vi "Determine Warnings.vi"() -> ()   [LabVIEW 2014]
panel:
  out "Warning Text":string
  out "Warning?":bool
  in  "Mininum Min Temp":dbl
  in  "Max Temp":dbl
  in  "Current Temp":dbl
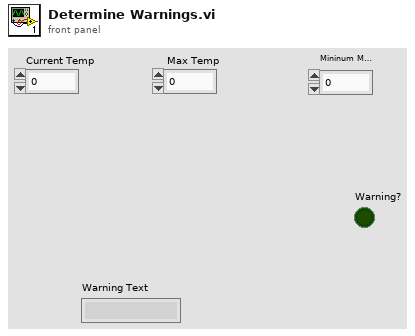
[diagram p1: front panel]
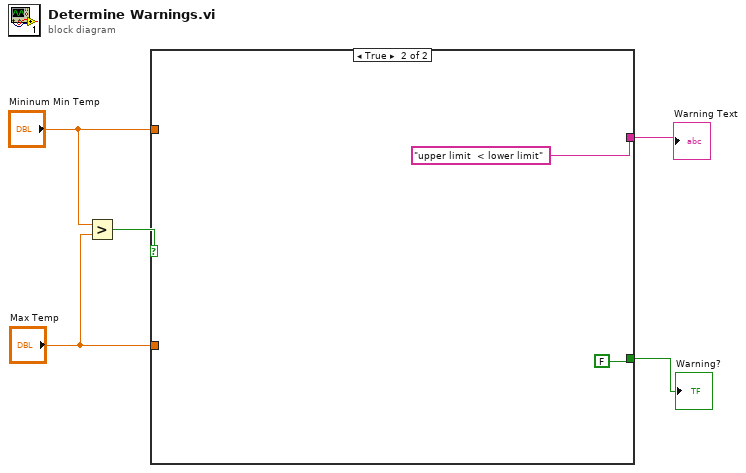
[diagram p0: block diagram]
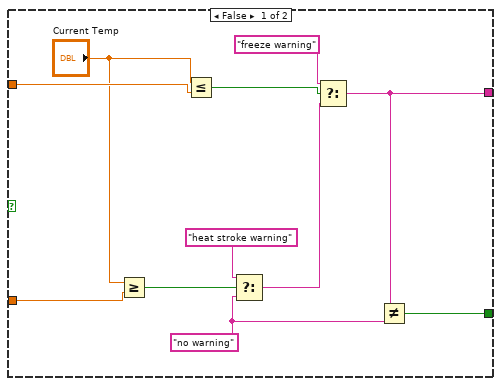
[diagram p2: hidden frame]
diagram:
  n1 = Greater?(x="Mininum Min Temp", y="Max Temp") -> (0:w3:bool)
  n2 = case shown="True" w3 {
    tunnel: "Mininum Min Temp" -> [w16 _]
    tunnel: "Max Temp" -> [w15 _]
    tunnel: [w8 "upper limit  < lower limit"] -> w2
    tunnel: [w6 FALSE] -> w1
    frame False {
      w7 = "no warning"
      n3 = Greater Or Equal?(x="Current Temp", y=w15) -> (x >= y?=w13:bool)
      n4 = Less Or Equal?(x="Current Temp", y=w16) -> (x <= y?=w11:bool)
      n5 = Select(t="heat stroke warning", s=w13, f=w7) -> (s? t:f=w9:string)
      n6 = Select(t="freeze warning", s=w11, f=w9) -> (s? t:f=w8:string)
      n7 = Not Equal?(x=w8, y=w7) -> (x != y?=w6:bool)
    }
    frame True {
    }
  }
  "Warning Text" <- w2
  "Warning?" <- w1
